vi "Get Channel Status.vi"(5 "Channel":i32=1 min=1 max=2 step=1, 7 "Slave":i32=1 min=1 max=6 step=1, 8 "error in (no error)":errorcluster, 11 "VISA resource name":refnum<visa-resource-name>) -> (0 "error out":errorcluster, 2 "Channel Enabled":bool, 3 "VISA resource name out":refnum<visa-resource-name>)   [LabVIEW 2020, in "QuPMXdriver.lvlib"]
doc: "Returns status of channel."
uses:
  QuPMXdriver.lvlib
  <vilib>/Utility/error.llb/Error Cluster From Error Code.vi
  <vilib>/ErrorRing/Error Ring.xnode
panel:
  out "read buffer":string="SLV SL%d CH%d "
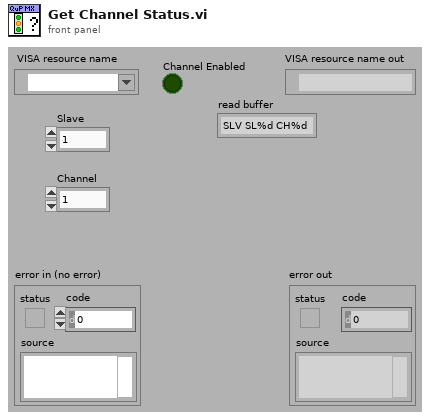
[diagram p1: front panel]
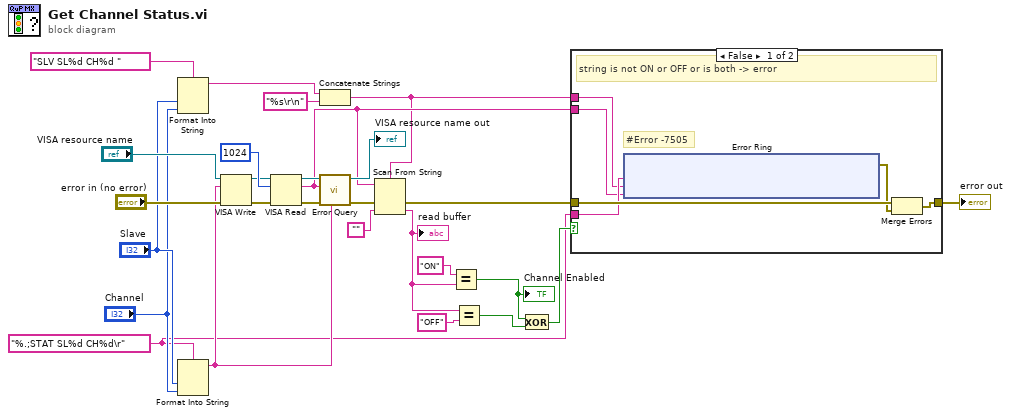
[diagram p0: block diagram]
diagram:
  w5 = "%.;STAT SL%d CH%d\r" ("format string")
  n1 = Format Into String(format string="SLV SL%d CH%d " ("read buffer"), "Slave", "Channel") -> (resulting string=w15:string)  [unwired: 2 in, 1 out]
  n2 = Format Into String(format string=w5, "Slave", "Channel") -> (resulting string=w20:string)  [unwired: 2 in, 1 out]
  n3 = VISA Write(VISA resource name="VISA resource name", write buffer=w20, error in (no error)="error in (no error)") -> (VISA resource name out=w22:refnum<visa-resource-name>, error out=w2:errorcluster)  [unwired: 1 out]
  n4 = VISA Read(VISA resource name=w22, byte count=u32 1024, error in (no error)=w2) -> (VISA resource name out=w23:refnum<visa-resource-name>, read buffer=w4:string, error out=w21:errorcluster)  [unwired: 1 out]
  n5 = Concatenate Strings(w15, "%s\r\n" ("read buffer")) -> (w3:string)
  n6 = call "Error Query.vi"("Last command"=w20, "error in (no error)"=w21, "Read buffer"=w4, "VISA resource name"=w23) -> ("error out"=w19:errorcluster, "VISA resource name out"=→"VISA resource name out":refnum<visa-resource-name>)  [unwired: 6 in]
  n7 = Scan From String(format string=w3, input string=w4, error in=w19, default 1="") -> (error out=w7:errorcluster, output 1=w13:string)  [unwired: 1 in, 2 out]
  "read buffer" <- w13
  n8 = Equal?(x="ON", y=w13) -> (x = y?=w6:bool)
  "Channel Enabled" <- w6
  n9 = Equal?(x=w13, y="OFF") -> (x = y?=w10:bool)
  n10 = Exclusive Or(1:w10, 2:w6) -> (0:w9:bool)
  n11 = case shown="False" w9 {
    tunnel: [w32 w43] -> w8
    tunnel: w7 -> [w33 w43]
    tunnel: w5 -> [w30 _]
    tunnel: w4 -> [w29 _]
    tunnel: w3 -> [w28 _]
    frame False {
      # "#Error -7505"
      # "string is not ON or OFF or is both -> error"
      n12 = xnode "Error Ring"("parameter 0"=w30, "parameter 1"=w28, "parameter 2"=w29) -> ("error out"=w31:errorcluster)
      n13 = Merge Errors(w33, w31) -> (w32:errorcluster)
    }
    frame True {
    }
  }
  "error out" <- w8
